vi "Basic Interface.vi"() -> ()   [LabVIEW 2018]
panel:
  in  "Read":bool
  out "Ready":bool
  in  "VISA resource name":refnum<visa-resource-name>
  out "read buffer 2":string
  in  "ms to wait":u32=1000
  out "return count of read":u32
  out "Busy":bool
  in  "stop":bool
  in  "Write":bool
  in  "write buffer":string="VER"
  out "error out":errorcluster
  out "read buffer":string
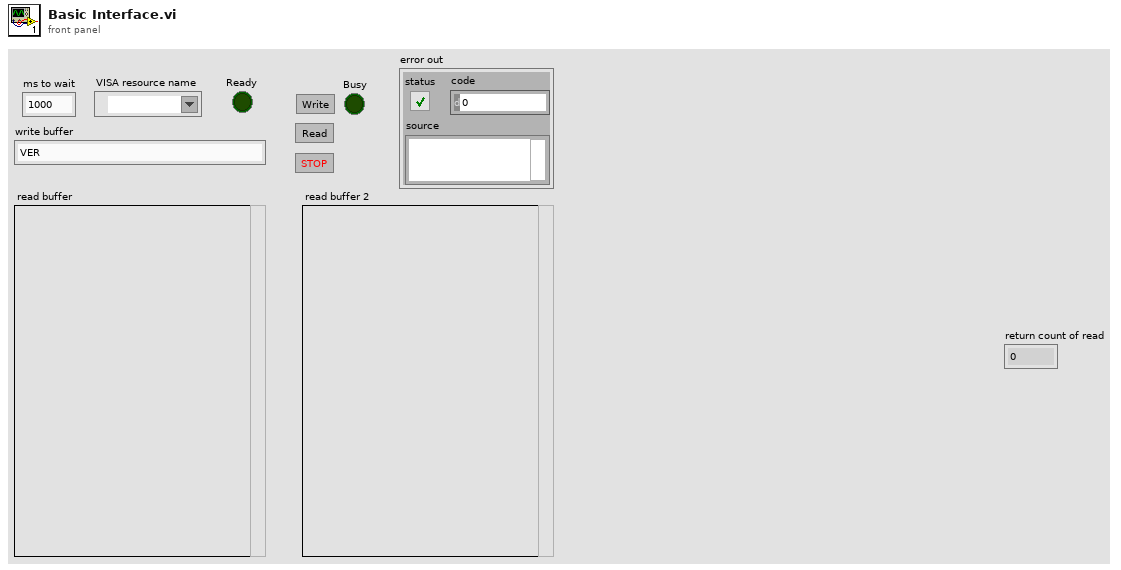
[diagram p1: front panel]
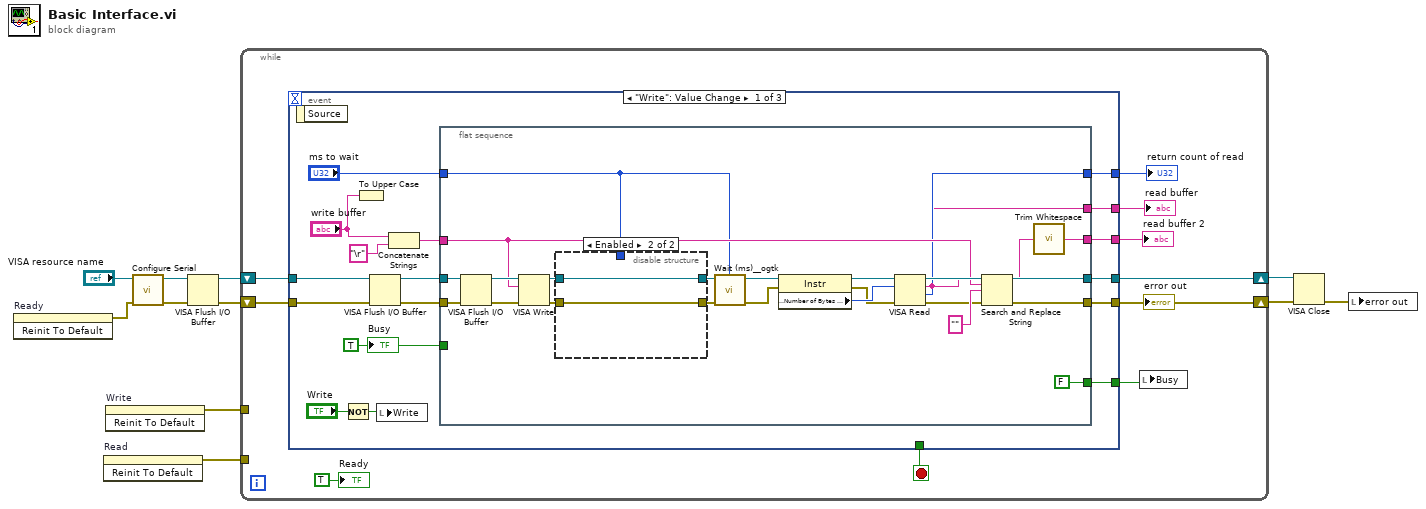
[diagram p0: block diagram]
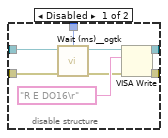
[diagram p2: hidden frame]
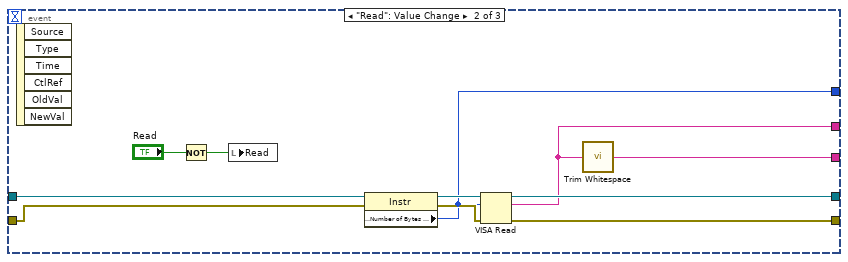
[diagram p3: hidden frame]
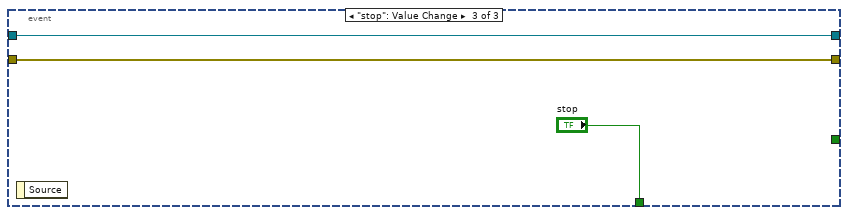
[diagram p4: hidden frame]
diagram:
  n1 = invoke on="Ready" class="Bool (strict)" method="Reinit To Default"() -> (error out=w2:errorcluster)  [unwired: 3 in, 2 out]
  n2 = invoke on="Read" class="Bool (strict)" method="Reinit To Default"() -> (error out=w1:errorcluster)  [unwired: 3 in, 2 out]
  n3 = invoke on="Write" class="Bool (strict)" method="Reinit To Default"() -> (error out=w3:errorcluster)  [unwired: 3 in, 2 out]
  n4 = call "Configure Serial.vi"("error in"=w2, "Resource Name"="VISA resource name") -> ("error out"=w7:errorcluster, "VISA out"=w8:refnum<visa-resource-name>)  [unwired: 8 in]
  n5 = VISA Flush I/O Buffer(VISA resource name=w8, error in (no error)=w7) -> (VISA resource name out=w5:refnum<visa-resource-name>, error out=w6:errorcluster)  [unwired: 1 in]
  n6 = while {
    shift-right: [w19] -> w11
    shift-left: w5 -> [w21]
    shift-right: [w12] -> w10
    shift-left: w6 -> [w20]
    tunnel: w3 -> [_]
    tunnel: w1 -> [_]
    stop <- w18 stop-if-true
    n7 = event shown="[0] \"Write\": Value Change" {
      selector: _ -> [_ _ _]
      dyn-events: _ -> [_ _ _]
      timeout: _ -> [_ _ _]
      tunnel: w21 -> [w26 w81 w83]
      tunnel: w20 -> [w25 w78 w82]
      tunnel: [w38 w79 w83] -> w19
      tunnel: [w37 w76 w82] -> w12
      tunnel: [_ _ "stop"] -> w18
      tunnel: [w30 _ _] -> w16
      tunnel: [w29 w75 _] -> w13
      tunnel: [w28 w73 _] -> w15
      tunnel: [w27 w74 _] -> w14
      event "Write": Value Change {
        w36 = TRUE ("Writing")
        n8 = event-data() -> ()  [unwired: 1 in, 1 out]
        n9 = Not(x="Write") -> (.not. x?=w32:bool)
        n10 = To Upper Case(1:"write buffer") -> ()  [unwired: 1 out]
        n11 = VISA Flush I/O Buffer(VISA resource name=w26, error in (no error)=w25) -> (VISA resource name out=w23:refnum<visa-resource-name>, error out=w24:errorcluster)  [unwired: 1 in]
        n12 = local write "Write"(w32) -> ()
        n13 = Concatenate Strings("write buffer", "\r" ("string")) -> (w34:string)
        n14 = flat-sequence {
          tunnel: [w60] -> w38
          tunnel: [w49] -> w37
          tunnel: [FALSE ("Writing")] -> w30
          tunnel: w23 -> [w55]
          tunnel: w24 -> [w54]
          tunnel: w36 -> [_]
          tunnel: w34 -> [w44]
          tunnel: "ms to wait" -> [w43]
          tunnel: [w39] -> w29
          tunnel: [w42] -> w28
          tunnel: [w41] -> w27
          frame #0 {
            n15 = VISA Flush I/O Buffer(VISA resource name=w55, error in (no error)=w54) -> (VISA resource name out=w52:refnum<visa-resource-name>, error out=w53:errorcluster)  [unwired: 1 in]
            n16 = VISA Write(VISA resource name=w52, write buffer=w44, error in (no error)=w53) -> (VISA resource name out=w48:refnum<visa-resource-name>, error out=w61:errorcluster)  [unwired: 1 out]
            n17 = disable-structure shown="Enabled" {
              disable-tunnel: w61 -> [w68 w69]
              disable-tunnel: w48 -> [w66 w70]
              disable-tunnel: [w65 w70] -> w47
              disable-tunnel: [w63 w69] -> w46
              disable-tunnel: w43 -> [w62 _]
              frame Disabled {
                n18 = call <userlib>:"Wait (ms)__ogtk.vi"("error in (no error)"=w68, "milliseconds to wait"=w62) -> ("error out"=w64:errorcluster)  [unwired: 8 in, 1 out]
                n19 = VISA Write(VISA resource name=w66, write buffer="R E DO16\r" ("string"), error in (no error)=w64) -> (VISA resource name out=w65:refnum<visa-resource-name>, error out=w63:errorcluster)  [unwired: 1 out]
              }
              frame Enabled {
              }
            }
            n20 = call <userlib>:"Wait (ms)__ogtk.vi"("error in (no error)"=w46, "milliseconds to wait"=w43) -> ("error out"=w45:errorcluster)  [unwired: 8 in, 1 out]
            n21 = property class="Instr"(reference=w47, error in=w45) -> (reference out=w58:refnum<visa-resource-name>, error out=w56:errorcluster, "Serial Settings:Number of Bytes at Serial Port"=w57:u32)
            n22 = VISA Read(VISA resource name=w58, byte count=w57, error in (no error)=w56) -> (VISA resource name out=w60:refnum<visa-resource-name>, read buffer=w41:string, return count=w42:u32, error out=w50:errorcluster)
            n23 = Search and Replace String(input string=w41, search string=w44, replace string="" ("replace string (\"\")"), error in=w50) -> (result string=w40:string, error out=w49:errorcluster)  [unwired: 4 in, 2 out]
            n24 = call <vilib>:"Trim Whitespace.vi"("string"=w40) -> ("trimmed string"=w39:string)  [unwired: 1 in]
          }
        }
        "Busy" <- w36
      }
      event "Read": Value Change {
        n25 = event-data() -> ()  [unwired: 1 in, 6 out]
        n26 = Not(x="Read") -> (.not. x?=w71:bool)
        n27 = local write "Read"(w71) -> ()
        n28 = property class="Instr"(reference=w81, error in=w78) -> (reference out=w80:refnum<visa-resource-name>, error out=w77:errorcluster, "Serial Settings:Number of Bytes at Serial Port"=w73:u32)
        n29 = VISA Read(VISA resource name=w80, byte count=w73, error in (no error)=w77) -> (VISA resource name out=w79:refnum<visa-resource-name>, read buffer=w74:string, error out=w76:errorcluster)  [unwired: 1 out]
        n30 = call <vilib>:"Trim Whitespace.vi"("string"=w74) -> ("trimmed string"=w75:string)  [unwired: 1 in]
      }
      event "stop": Value Change {
        n31 = event-data() -> ()  [unwired: 1 in, 1 out]
      }
    }
    "read buffer 2" <- w13
    "read buffer" <- w14
    "return count of read" <- w15
    "error out" <- w12
    n32 = local write "Busy"(w16) -> ()
    "Ready" <- TRUE ("Ready")
  }
  n33 = VISA Close(VISA resource name=w11, error in (no error)=w10) -> (error out=w9:errorcluster)
  n34 = local write "error out"(w9) -> ()
